vi "parseAzimuthPositionShortStatus.vi"(8 "error in (no error)":errorcluster, 10 "shortStatus":string, 11 "DomeCommunicator in":refnum<class "ATDomeCommunicator.lvclass">) -> (0 "error out":errorcluster, 1 "azimuth":dbl, 2 "domePosition":T1, 3 "DomeCommunicator out":refnum<class "ATDomeCommunicator.lvclass">)   [LabVIEW 2016, in "ATDomeCommunicator.lvclass"]
uses:
  ATDomeCommunicator.lvclass
  ComTypedefs/azimimuthPositionStatus.ctl
  IDome/domeTypedefs/azimuth.ctl
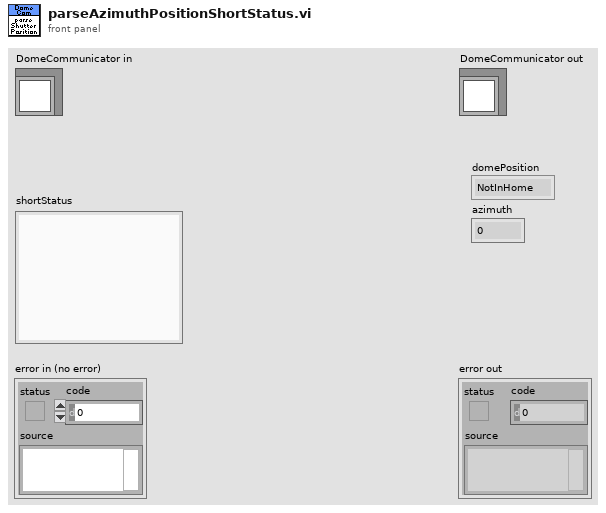
[diagram p1: front panel]
types:
  T1 = typedef "azimimuthPositionStatus.ctl" = enum16{"NotInHome", "Home"}
  T2 = typedef "azimuth.ctl" = dbl
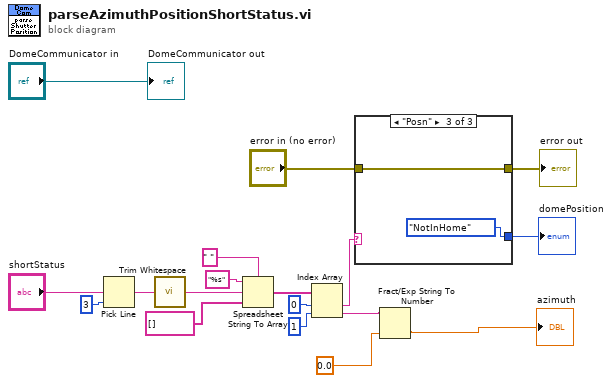
[diagram p0: block diagram]
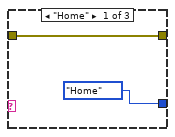
[diagram p2: hidden frame]
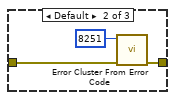
[diagram p3: hidden frame]
diagram:
  n1 = Pick Line(multi-line string="shortStatus", line index=3) -> (output string=w16:string)  [unwired: 1 in]
  n2 = call <vilib>:"Trim Whitespace.vi"("string"=w16) -> ("trimmed string"=w11:string)  [unwired: 1 in]
  n3 = Spreadsheet String To Array(delimiter (Tab)=" ", format string="%s", spreadsheet string=w11, array type (2D Dbl)=string[] []) -> (array=w7:string[])
  n4 = Index Array(array=w7, index #1=0 ("index"), index #2=1 ("index")) -> (element #1=w5:string, element #2=w3:string)
  n5 = case shown="\"Posn\"" w5 {
    tunnel: "error in (no error)" -> [w20 w22 w25]
    tunnel: [w20 w23 w25] -> w10
    tunnel: [azimimuthPositionStatus."Home" ("domePosition") _ azimimuthPositionStatus."NotInHome" ("domePosition")] -> w4
    frame "Home" {
    }
    frame Default {
      n6 = call <vilib>:"Error Cluster From Error Code.vi"("error in (no error)"=w22, "error code (0)"=8251) -> ("error out"=w23:errorcluster)  [unwired: 7 in]
    }
    frame "Posn" {
    }
  }
  "error out" <- w10
  "domePosition" <- w4
  n7 = Fract/Exp String To Number(string=w3, default (0 dbl)=T2 0.0 ("azimuth")) -> (number=→"azimuth":dbl)  [unwired: 2 in, 1 out]
  "DomeCommunicator out" <- "DomeCommunicator in"
